vi "global variable.vi"() -> ()   [LabVIEW 2014]
panel:
  out "状态显示":string
  in  "屏蔽":bool
  out "Reject":dbl
  out "BST(%)":dbl format="%.1f%%"
  out "型号":string
  in  "数值":dbl
  in  "每小时FTT":dbl[](array[numeric])
  in  "每小时产量":dbl[](array[numeric])
  out "产线名称":string
  out "FTT Rate":dbl format="%.1f%%"
  out "FTT":dbl
  out "Repair":dbl
  out "Done":dbl
  out "Actual":dbl
  out "Plan":dbl
  out "Rate":dbl format="%.1f%%"
  out "Target":dbl
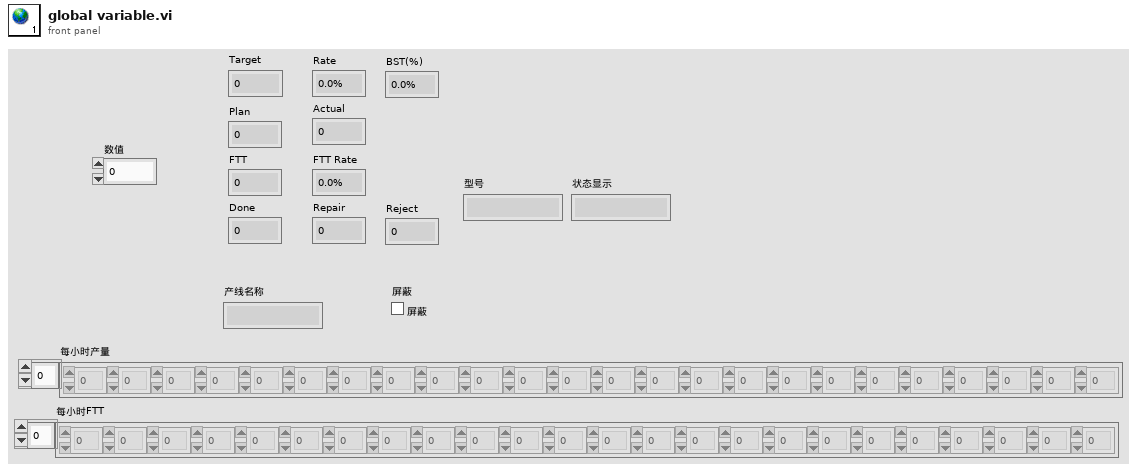
[diagram p1: front panel]
diagram:
